vi "Diagramme de Bode pour Labview salle JPB.vi"() -> ()   [LabVIEW 2024]
doc: "This VI simulates an application that uses GPIB instruments to perform a frequency response test on a unit under test(UUT). A function generator supplies a sinusoidal input to the UUT (a bandpass filter in this example), and a digital multimeter measures the output voltage of the UUT. \n\nThe LabVIEW concepts of the For Loop, the Formula Node, the graph, and arrays are shown in this example."
panel:
  out "frequence de coupure":dbl
  out "indice fractionaire":dbl
  out "Gain -3B":dbl
  out "Numérique":dbl
  in  "Waveform":enum16{"SIN", "TRI", "SQR"}(ring)
  out "freq":dbl(knob) scale=0.0..10000.0
  out "Tension":string
  in  "VISA GPIB  Agient":refnum<visa-resource-name>="GPIB0::2::INSTR" caption="Ressource GPIB VISA"
  in  "Agilent":string
  in  "VISA GPIB Resource":refnum<visa-resource-name>="GPIB0::2::INSTR" caption="Ressource GPIB VISA"
  in  "Number of Steps":dbl(knob)=10.0 scale=0.0..10.0
  in  "Fréquence haute":dbl(knob)=10000.0 scale=0.0..10.0
  in  "Fréquence basse":dbl(knob)=1.0 scale=0.0..10.0
  in  "Amplitude":dbl(knob)=1.0 scale=0.0..10.0
  out "Graphe":cluster{dbl[], dbl[]}(graph)
  # "Amplitude"
  # "Nombre de pas"
  # "Fréquence basse"
  # "Fréquence haute"
  # "Réponse fréquentielle"
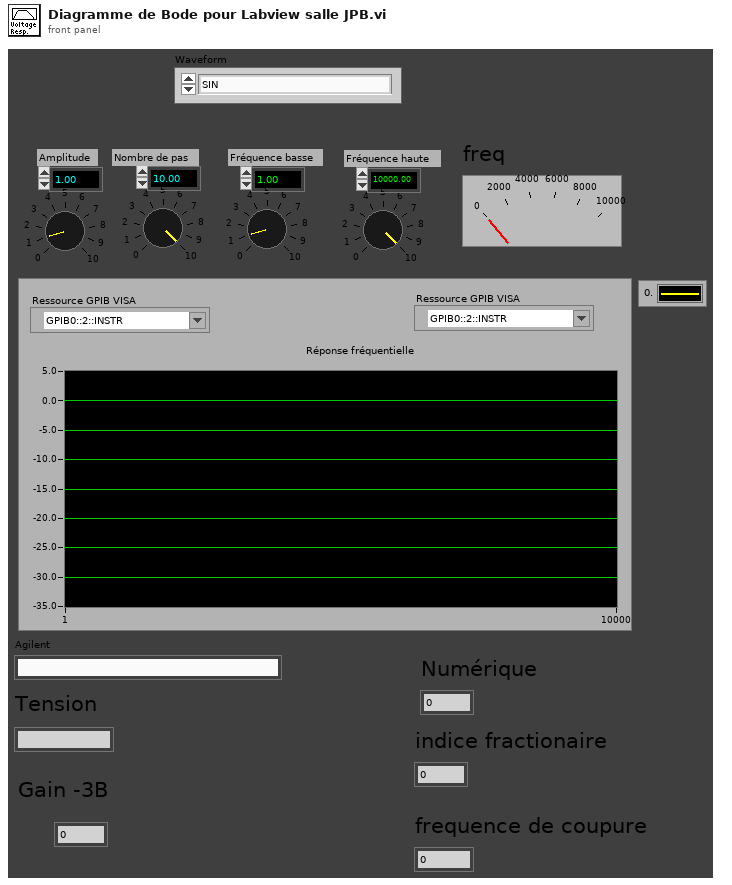
[diagram p1: front panel]
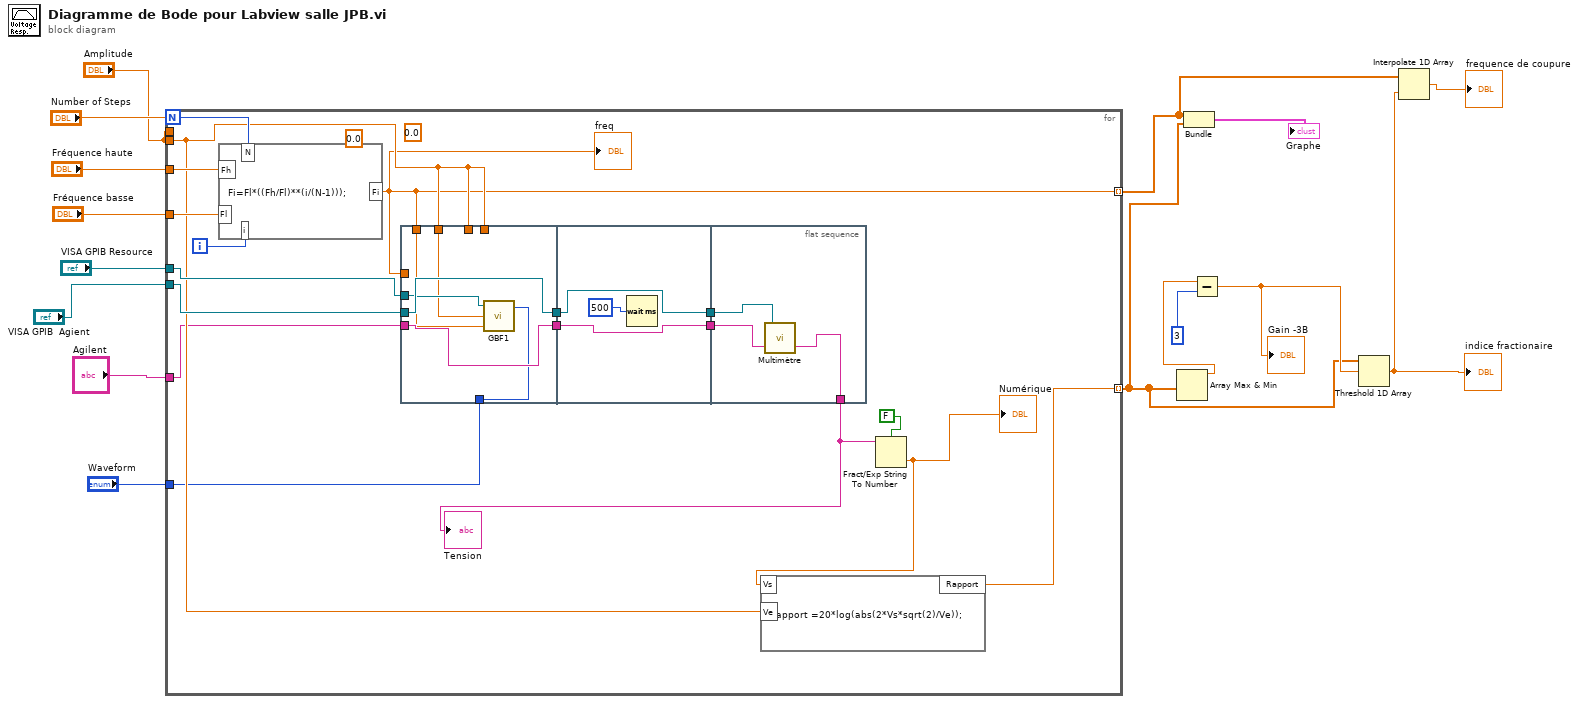
[diagram p0: block diagram]
diagram:
  n1 = for {
    N: "Number of Steps" -> [w34]
    tunnel: "Amplitude" -> [w27]
    tunnel: "Fréquence basse" -> [w32]
    tunnel: "Fréquence haute" -> [w33]
    tunnel: [w25] -> w3 mode=indexing
    tunnel: "VISA GPIB Resource" -> [w30]
    tunnel: "Amplitude" -> [_]
    tunnel: "Agilent" -> [w26]
    tunnel: [w29] -> w4 mode=indexing
    tunnel: "VISA GPIB  Agient" -> [w28]
    tunnel: "Waveform" -> [w17]
    i -> [w31]
    (unwired) 0.0 ("Numérique")
    (unwired) 0.0 ("Numérique")
    n2 = formula code="Fi=Fl*((Fh/Fl)**(i/(N-1)));"("N"=w34, "Fh"=w33, "Fl"=w32, "i"=w31) -> ("Fi"=w25:dbl)
    "freq" <- w25
    n3 = flat-sequence {
      tunnel: w30 -> [w38]
      tunnel: w27 -> [_]
      tunnel: w25 -> [_]
      tunnel: w27 -> [_]
      tunnel: w28 -> [w39]
      tunnel: [w39] -> w21
      tunnel: w27 -> [w35]
      tunnel: w26 -> [w40]
      tunnel: [w40] -> w20
      tunnel: w25 -> [w37]
      tunnel: w17 -> [w36]
      tunnel: w21 -> [w42]
      tunnel: [w42] -> w19
      tunnel: w20 -> [w41]
      tunnel: [w41] -> w18
      tunnel: w19 -> [w46]
      tunnel: w18 -> [w45]
      tunnel: [w44] -> w24
      frame #0 {
        n4 = call "GBF1.vi"("Waveform"=w36, "Fréquence"=w37, "Amplitude"=w35, "Ressource GPIB VISA"=w38) -> ()  [unwired: 2 in]
      }
      frame #1 {
        n5 = Wait (ms)(milliseconds to wait=500) -> ()  [unwired: 1 out]
      }
      frame #2 {
        n6 = call "Multimètre.vi"("Commande"=w45, "Ressource GPIB VISA"=w46) -> ("tension en chaine de caractères"=w44:string)  [unwired: 1 in]
      }
    }
    n7 = Fract/Exp String To Number(use system decimal point (T)=FALSE, string=w24) -> (number=w23:dbl)  [unwired: 2 in, 1 out]
    "Numérique" <- w23
    n8 = formula code="Rapport =20*log(abs(2*Vs*sqrt(2)/Ve));"("Vs"=w23, "Ve"=w27) -> ("Rapport"=w29:dbl)
    "Tension" <- w24
  }
  n9 = Array Max & Min(array=w4) -> (max value=w6:dbl)  [unwired: 3 out]
  n10 = Bundle(w3, w4) -> (→"Graphe":cluster{dbl[], dbl[]})  [unwired: 1 in]
  n11 = Subtract(x=w6, y=3) -> (x-y=w5:dbl)
  "Gain -3B" <- w5
  n12 = Threshold 1D Array(2:w5, 3:w4) -> (0:w2:dbl)  [unwired: 1 in]
  "indice fractionaire" <- w2
  n13 = Interpolate 1D Array(1:w2, 2:w3) -> (0:→"frequence de coupure":dbl)
